vi "Main Engine Init Data Log File.vi"(8 "error in":errorcluster, 10 "PLL Status":string, 11 "Engine Name":string) -> (0 "error out":errorcluster, 2 "Log File Path":path)   [LabVIEW 2024]
doc: "All Rights Reserved © 2023 SyncSols"
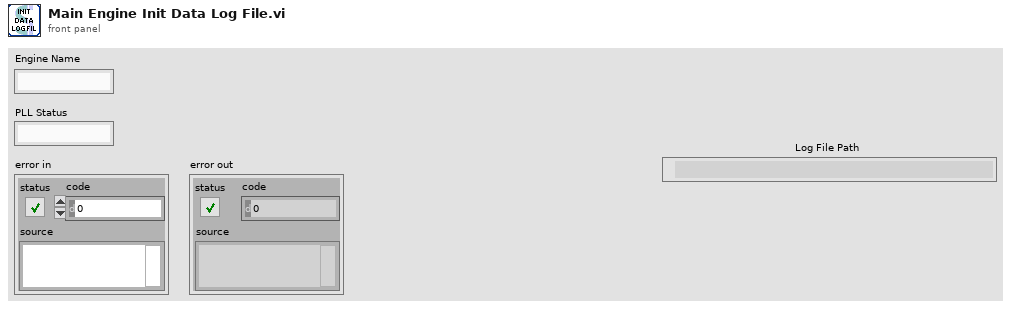
[diagram p1: front panel]
types:
  T1 = enum16{"open", "replace", "create", "open or create", "replace or create", "replace or create with confirmation"}
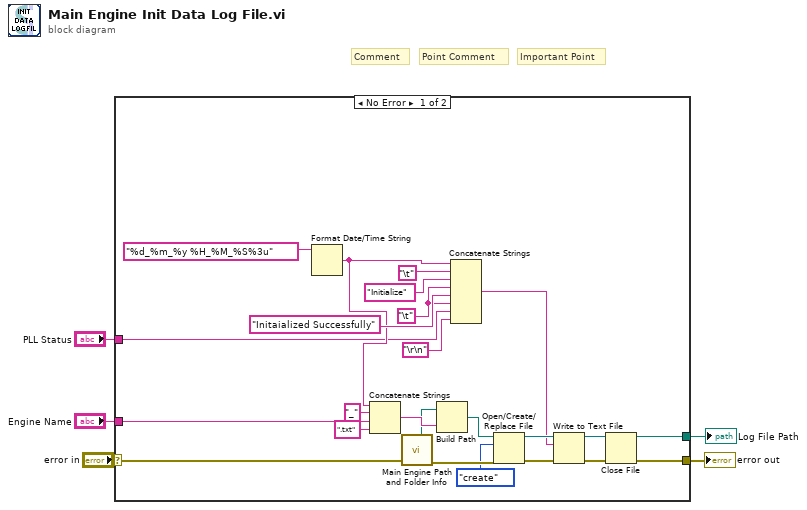
[diagram p0: block diagram]
diagram:
  # "Important Point"
  # "Point Comment"
  # "Comment"
  n1 = case shown="No Error" "error in" {
    selector: "error in" -> [w20 w30]
    tunnel: [w7 w30] -> w5
    tunnel: "Engine Name" -> [w18 _]
    tunnel: "PLL Status" -> [w11 _]
    tunnel: [w6 _] -> w1
    frame No Error {
      w12 = "\t"
      n2 = Format Date/Time String(time format string (%c)="%d_%m_%y %H_%M_%S%3u") -> (date/time string=w13:string)  [unwired: 2 in]
      n3 = Concatenate Strings(w13, "_" ("string"), w18, ".txt" ("string")) -> (w16:string)
      n4 = call "Main Engine Path and Folder Info.vi"("error in"=w20) -> ("error out"=w29:errorcluster, "Data Logging"=w10:path)  [unwired: 4 in, 5 out]
      n5 = Build Path(base path=w10, name or relative path=w16) -> (appended path=w28:path)
      n6 = Concatenate Strings(w13, "\t", "Initialize", w12, "Initaialized Successfully" ("string"), w12, w11, "\r\n") -> (w19:string)
      n7 = Open/Create/Replace File(file path (use dialog)=w28, error in=w29, operation (0:open)=T1."create") -> (refnum out=w25:refnum<file>, error out=w26:errorcluster)  [unwired: 3 in, 1 out]
      n8 = Write to Text File(file (use dialog)=w25, text=w19, error in=w26) -> (refnum out=w9:refnum<file>, error out=w8:errorcluster)  [unwired: 1 in, 1 out]
      n9 = Close File(refnum=w9, error in=w8) -> (path=w6:path, error out=w7:errorcluster)
    }
    frame Error {
    }
  }
  "error out" <- w5
  "Log File Path" <- w1
